vi "俄罗斯方块-绘制网格.vi"(0 "图片输入":picture, 1 "xN":i16=3, 2 "yN":i16=3, 3 "数组":u32[][](array[colorbox]), 5 "块边长":i32=35, 7 "边框色":u32(colorbox), 9 "线色":u32(colorbox)=13948116, 11 "画笔":T1={"Width"=1, "Style"=enum."Solid"}, 12 "xOffset":i16=366, 13 "yOffset":i16=504, 14 "消息文本":string, 15 "消息颜色":u32(colorbox)) -> (4 "图片输出":picture)   [LabVIEW 2016]
panel:
  out "topReal+LineWidth":u16
  out "leftReal+LineWidth":u16
  out "rightReal-LineWidth":i32
  out "bottomReal-LineWidth":i32
  out "LineWidth":u16
  out "bottomReal":i16
  out "rightReal":i16
  out "topReal":i16
  out "leftReal":i16
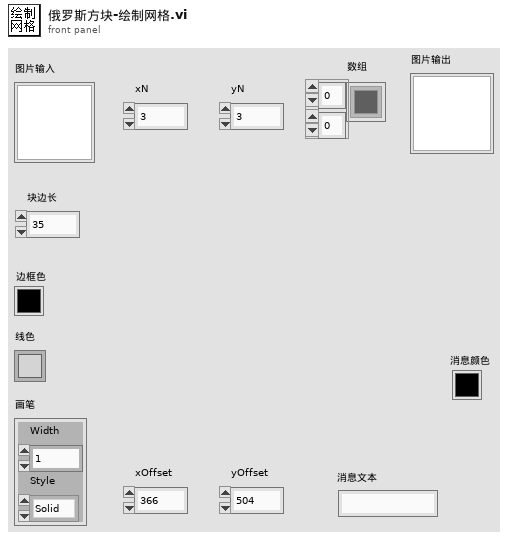
[diagram p1: front panel]
types:
  T1 = cluster{"Width":u16, "Style":enum32{"Solid", "Dash", "Dot", "DashDot", "DashDotDot"}}
  T2 = cluster{"Font Name:":string, "Size":i16, "Strikeout?":bool, "Italic?":bool, "Underline?":bool, "Outline?":bool, "Shadow?":bool, "Bold?":bool}
  T3 = cluster{"horizontal":enum16{"left", "center", "right"}, "vertical":enum16{"top", "center", "bottom"}}
  T4 = enum16{"User-specified Font", "Application Font", "System Font", "Dialog Font"}
  T5 = cluster{"leftReal":i16, "topReal":i16, "rightReal-LineWidth":i32, "bottomReal-LineWidth":i32}
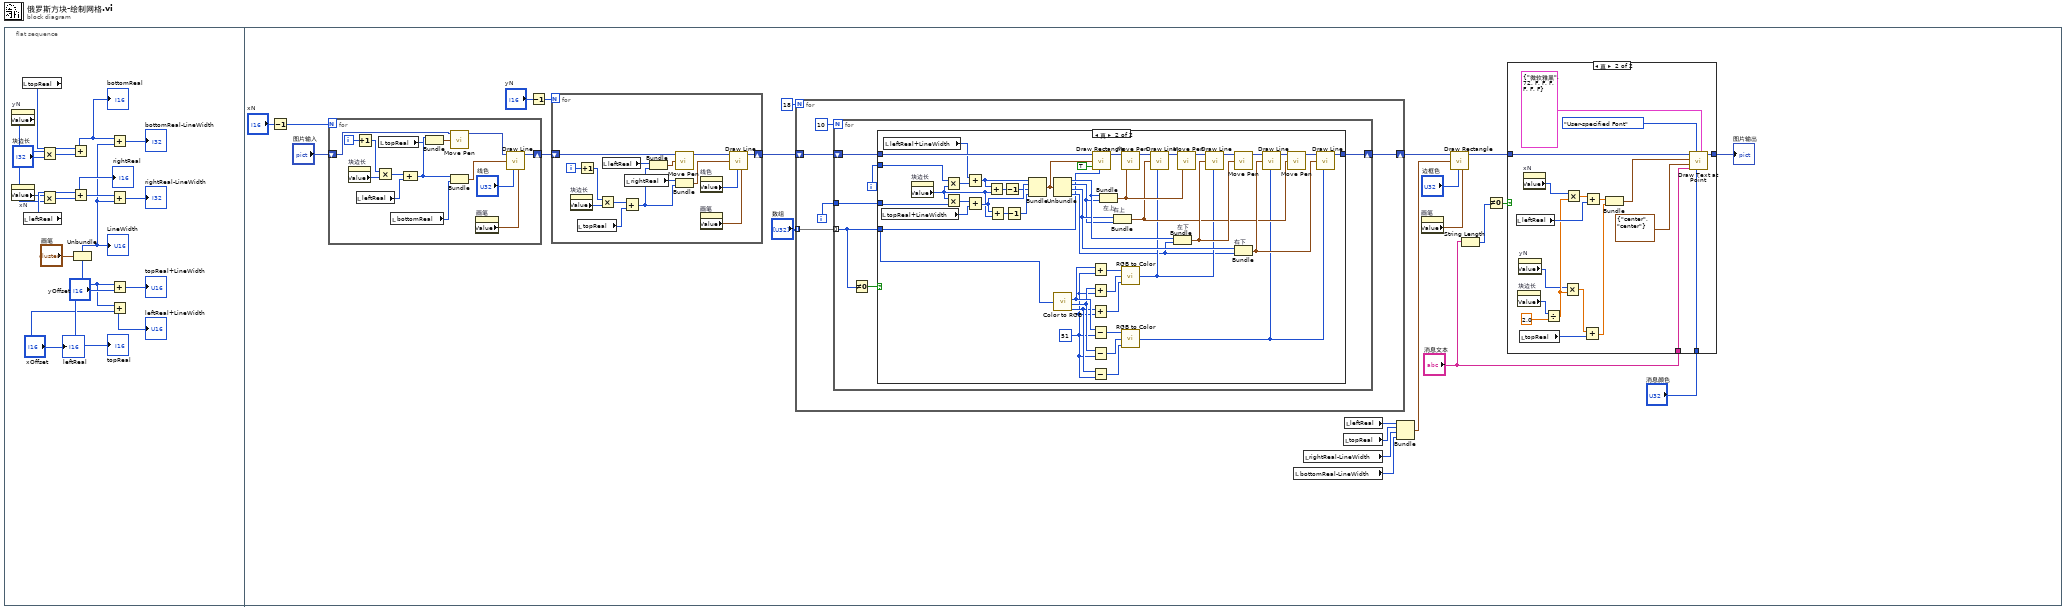
[diagram p0: block diagram]
diagram:
  n1 = flat-sequence {
    frame #0 {
      n2 = property on="yN" class="DigNum (严格)"() -> ("Value"=w11:i16)  [unwired: 2 in, 2 out]
      n3 = property on="xN" class="DigNum (严格)"() -> ("Value"=w12:i16)  [unwired: 2 in, 2 out]
      n4 = local read "topReal"() -> (w16:i16)
      n5 = local read "leftReal"() -> (w14:i16)
      n6 = Multiply(x=w11, y="块边长") -> (x*y=w17:i32)
      n7 = Multiply(x=w12, y="块边长") -> (x*y=w15:i32)
      n8 = Add(x=w16, y=w17) -> (x+y=w9:i32)
      "bottomReal" <- w9
      n9 = Add(x=w14, y=w15) -> (x+y=w7:i32)
      "rightReal" <- w7
      n10 = Unbundle("画笔") -> ("Width"=w2:u16)  [unwired: 1 out]
      "LineWidth" <- w2
      n11 = Add(x=w9, y=w2) -> (x+y=→"bottomReal-LineWidth":i32)
      n12 = Add(x=w7, y=w2) -> (x+y=→"rightReal-LineWidth":i32)
      n13 = Add(x=w2, y="yOffset") -> (x+y=→"topReal+LineWidth":u16)
      n14 = Add(x=w2, y="xOffset") -> (x+y=→"leftReal+LineWidth":u16)
      "leftReal" <- "xOffset"
      "topReal" <- "yOffset"
    }
    frame #1 {
      n15 = Decrement(x="xN") -> (x-1=w37:i16)
      n16 = for {
        N: w37 -> [_]
        shift-right: [w148] -> w40
        shift-left: "图片输入" -> [w146]
        i -> [w143]
        n17 = property on="块边长" class="DigNum (严格)"() -> ("Value"=w138:i32)  [unwired: 2 in, 2 out]
        n18 = Increment(x=w143) -> (x+1=w144:i32)
        n19 = local read "leftReal"() -> (w135:i16)
        n20 = Multiply(x=w144, y=w138) -> (x*y=w142:i32)
        n21 = local read "topReal"() -> (w136:i16)
        n22 = local read "bottomReal"() -> (w137:i16)
        n23 = Compound Arithmetic op=ADD(w142, w135) -> (w141:i32)
        n24 = Bundle(w141, "topReal"=w136) -> (w139:cluster{i32, "topReal":i16})  [unwired: 1 in]
        n25 = call <vilib>:"Move Pen.vi"("new position"=w139, "picture"=w146) -> ("new picture"=w147:picture)  [unwired: 3 in]
        n26 = Bundle(w141, "bottomReal"=w137) -> (w145:cluster{i32, "bottomReal":i16})  [unwired: 1 in]
        n27 = property on="画笔" class="Clust (严格)"() -> ("Value"=w134:T1)  [unwired: 2 in, 2 out]
        n28 = call <vilib>:"Draw Line.vi"("picture"=w147, "end point"=w145, "color(black)"="线色", "pen"=w134) -> ("new picture"=w148:picture)  [unwired: 5 in]
      }
      n29 = Decrement(x="yN") -> (x-1=w36:i16)
      n30 = for {
        N: w36 -> [_]
        shift-right: [w133] -> w25
        shift-left: w40 -> [w131]
        i -> [w127]
        n31 = property on="块边长" class="DigNum (严格)"() -> ("Value"=w124:i32)  [unwired: 2 in, 2 out]
        n32 = local read "topReal"() -> (w119:i16)
        n33 = Increment(x=w127) -> (x+1=w128:i32)
        n34 = Multiply(x=w128, y=w124) -> (x*y=w126:i32)
        n35 = local read "leftReal"() -> (w121:i16)
        n36 = Add(x=w126, y=w119) -> (x+y=w125:i32)
        n37 = local read "rightReal"() -> (w120:i16)
        n38 = Bundle("leftReal"=w121, w125) -> (w130:cluster{"leftReal":i16, i32})  [unwired: 1 in]
        n39 = call <vilib>:"Move Pen.vi"("new position"=w130, "picture"=w131) -> ("new picture"=w132:picture)  [unwired: 3 in]
        n40 = Bundle("rightReal"=w120, w125) -> (w129:cluster{"rightReal":i16, i32})  [unwired: 1 in]
        n41 = property on="线色" class="ColBox"() -> ("Value"=w123:u32)  [unwired: 2 in, 2 out]
        n42 = property on="画笔" class="Clust (严格)"() -> ("Value"=w122:T1)  [unwired: 2 in, 2 out]
        n43 = call <vilib>:"Draw Line.vi"("picture"=w132, "end point"=w129, "color(black)"=w123, "pen"=w122) -> ("new picture"=w133:picture)  [unwired: 5 in]
      }
      n44 = for {
        N: 18 -> [_]
        tunnel: "数组" -> [w64] mode=indexing
        shift-right: [w63] -> w26
        shift-left: w25 -> [w62]
        i -> [w61]
        n45 = for {
          N: 10 -> [_]
          tunnel: w64 -> [w68] mode=indexing
          shift-right: [w71] -> w63
          shift-left: w62 -> [w70]
          tunnel: w61 -> [w66]
          i -> [w67]
          n46 = Not Equal To 0?(x=w68) -> (x != 0?=w69:bool)
          n47 = case shown="真" w69 {
            tunnel: [w72 w100] -> w71
            tunnel: w70 -> [w72 w118]
            tunnel: w68 -> [_ w79]
            tunnel: w67 -> [_ w73]
            tunnel: w66 -> [_ w116]
            frame False {
            }
            frame True {
              w81 = u8 51
              n48 = local read "topReal+LineWidth"() -> (w113:u16)
              n49 = local read "leftReal+LineWidth"() -> (w114:u16)
              n50 = property on="块边长" class="DigNum (严格)"() -> ("Value"=w74:i32)  [unwired: 2 in, 2 out]
              n51 = Multiply(x=w73, y=w74) -> (x*y=w115:i32)
              n52 = Multiply(x=w74, y=w116) -> (x*y=w112:i32)
              n53 = Add(x=w114, y=w115) -> (x+y=w110:i32)
              n54 = Add(x=w112, y=w113) -> (x+y=w111:i32)
              n55 = Add(x=w110, y=w74) -> (x+y=w76:i32)
              n56 = Add(x=w111, y=w74) -> (x+y=w77:i32)
              n57 = Decrement(x=w76) -> (x-1=w75:i32)
              n58 = Decrement(x=w77) -> (x-1=w78:i32)
              n59 = Bundle(w110, w111, w75, w78) -> (w99:cluster{i32, i32, i32, i32})  [unwired: 1 in]
              n60 = Unbundle(w99) -> (w97:i32, w95:i32, w96:i32, w80:i32)
              n61 = call <vilib>:"Color to RGB.vi"("Color"=w79) -> ("R"=w84:u8, "G"=w83:u8, "B"=w82:u8)  [unwired: 1 out]
              n62 = Add(x=w84, y=w81) -> (x+y=w90:u8)
              n63 = Add(x=w83, y=w81) -> (x+y=w89:u8)
              n64 = Add(x=w82, y=w81) -> (x+y=w88:u8)
              n65 = Subtract(x=w84, y=w81) -> (x-y=w87:u8)
              n66 = Subtract(x=w83, y=w81) -> (x-y=w86:u8)
              n67 = Subtract(x=w82, y=w81) -> (x-y=w85:u8)
              n68 = call <vilib>:"Draw Rectangle.vi"("picture"=w118, "rect"=w99, "fill?(F)"=TRUE, "color(black)"=w79) -> ("new picture"=w109:picture)  [unwired: 5 in]
              n69 = Bundle "左上"(w97, w95) -> (w107:cluster{i32, i32})  [unwired: 1 in]
              n70 = Bundle "右上"(w96, w95) -> (w93:cluster{i32, i32})  [unwired: 1 in]
              n71 = call <vilib>:"RGB to Color.vi"("B"=w88, "G"=w89, "R"=w90) -> ("Color"=w92:u32)
              n72 = call <vilib>:"RGB to Color.vi"("B"=w85, "G"=w86, "R"=w87) -> ("Color"=w91:u32)
              n73 = call <vilib>:"Move Pen.vi"("new position"=w107, "picture"=w109) -> ("new picture"=w108:picture)  [unwired: 3 in]
              n74 = call <vilib>:"Draw Line.vi"("picture"=w108, "end point"=w93, "color(black)"=w92) -> ("new picture"=w106:picture)  [unwired: 6 in]
              n75 = Bundle "左下"(w97, w80) -> (w94:cluster{i32, i32})  [unwired: 1 in]
              n76 = call <vilib>:"Move Pen.vi"("new position"=w107, "picture"=w106) -> ("new picture"=w105:picture)  [unwired: 3 in]
              n77 = call <vilib>:"Draw Line.vi"("picture"=w105, "end point"=w94, "color(black)"=w92) -> ("new picture"=w104:picture)  [unwired: 6 in]
              n78 = call <vilib>:"Move Pen.vi"("new position"=w94, "picture"=w104) -> ("new picture"=w103:picture)  [unwired: 3 in]
              n79 = Bundle "右下"(w96, w80) -> (w98:cluster{i32, i32})  [unwired: 1 in]
              n80 = call <vilib>:"Draw Line.vi"("picture"=w103, "end point"=w98, "color(black)"=w91) -> ("new picture"=w102:picture)  [unwired: 6 in]
              n81 = call <vilib>:"Move Pen.vi"("new position"=w93, "picture"=w102) -> ("new picture"=w101:picture)  [unwired: 3 in]
              n82 = call <vilib>:"Draw Line.vi"("picture"=w101, "end point"=w98, "color(black)"=w91) -> ("new picture"=w100:picture)  [unwired: 6 in]
            }
          }
        }
      }
      n83 = local read "bottomReal-LineWidth"() -> (w31:i32)
      n84 = local read "rightReal-LineWidth"() -> (w32:i32)
      n85 = local read "topReal"() -> (w33:i16)
      n86 = local read "leftReal"() -> (w34:i16)
      n87 = Bundle("leftReal"=w34, "topReal"=w33, "rightReal-LineWidth"=w32, "bottomReal-LineWidth"=w31) -> (w22:T5)  [unwired: 1 in]
      n88 = property on="画笔" class="Clust (严格)"() -> ("Value"=w38:T1)  [unwired: 2 in, 2 out]
      n89 = call <vilib>:"Draw Rectangle.vi"("picture"=w26, "rect"=w22, "color(black)"="边框色", "pen"=w38) -> ("new picture"=w24:picture)  [unwired: 5 in]
      n90 = String Length(string="消息文本") -> (length=w21:i32)
      n91 = Not Equal To 0?(x=w21) -> (x != 0?=w19:bool)
      n92 = case shown="真" w19 {
        tunnel: w24 -> [w41 w60]
        tunnel: [w41 w59] -> w23
        tunnel: "消息文本" -> [_ w43]
        tunnel: "消息颜色" -> [_ w42]
        frame False {
        }
        frame True {
          n93 = local read "leftReal"() -> (w55:i16)
          n94 = property on="块边长" class="DigNum (严格)"() -> ("Value"=w48:i32)  [unwired: 2 in, 2 out]
          n95 = property on="yN" class="DigNum (严格)"() -> ("Value"=w45:i16)  [unwired: 2 in, 2 out]
          n96 = local read "topReal"() -> (w51:i16)
          n97 = property on="xN" class="DigNum (严格)"() -> ("Value"=w44:i16)  [unwired: 2 in, 2 out]
          n98 = Divide(x=w48, y=2.0) -> (x/y=w46:dbl)
          n99 = Multiply(x=w45, y=w46) -> (x*y=w52:dbl)
          n100 = Multiply(x=w44, y=w46) -> (x*y=w54:dbl)
          n101 = Add(x=w52, y=w51) -> (x+y=w50:dbl)
          n102 = Add(x=w54, y=w55) -> (x+y=w53:dbl)
          n103 = Bundle(w53, w50) -> (w56:cluster{dbl, dbl})  [unwired: 1 in]
          n104 = call <vilib>:"Draw Text at Point.vi"("[user-specified font]"=T2 {"Font Name:"="微软雅黑", "Size"=72, "Strikeout?"=FALSE, "Italic?"=FALSE, "Underline?"=FALSE, "Outline?"=FALSE, "Shadow?"=FALSE, "Bold?"=FALSE}, "text color(black)"=w42, "desired font(Application)"=T4."User-specified Font", "text"=w43, "alignment(left, top)"=T3 {"horizontal"=enum."center", "vertical"=enum."center"}, "origin"=w56, "picture"=w60) -> ("new picture"=w59:picture)  [unwired: 3 in, 1 out]
        }
      }
      "图片输出" <- w23
    }
  }
